vi "Set Modulation Mode.vi"(8 "error in (no error)":errorcluster, 9 "Modulation Mode (def: AM)":u16(ring)=1 items=["n/a", "AM", "FM", "PM", "FSK", "PWM"], 10 "Channel (0: Channel 1)":T1 items=["Channel 1", "Channel 2"], 11 "VISA resource name":refnum<visa-resource-name>) -> (0 "error out":errorcluster, 3 "VISA resource name out":refnum<visa-resource-name>)   [LabVIEW 2017, in "Tektronix AFG 3000 Series.lvlib"]
doc: "If pulse waveform and something other than PWM is desired, it will set the waveform to sine."
uses:
  Tektronix AFG 3000 Series.lvlib
  controls.llb/Channel.ctl
  controls.llb/Waveform Shape.ctl
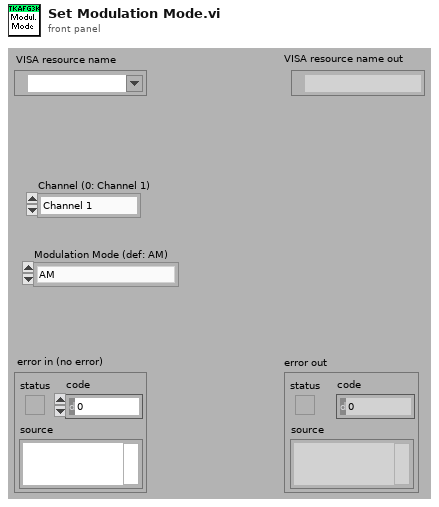
[diagram p1: front panel]
types:
  T1 = typedef "Channel.ctl" = u16
  T2 = typedef "Waveform Shape.ctl" = u16
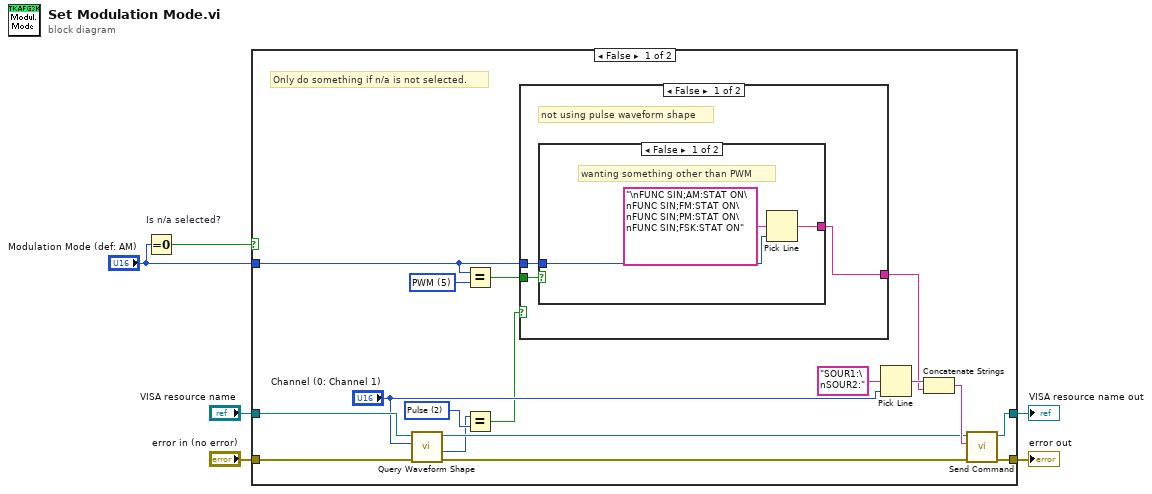
[diagram p0: block diagram]
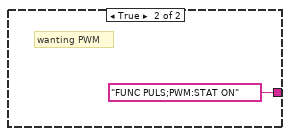
[diagram p2: hidden frame]
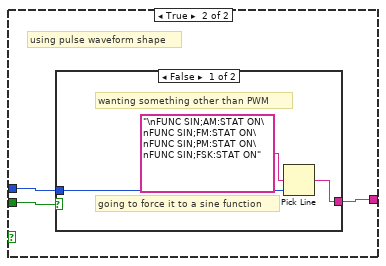
[diagram p3: hidden frame]
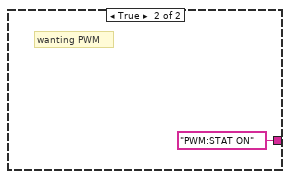
[diagram p4: hidden frame]
diagram:
  n1 = Equal To 0? "Is n/a selected?"(x="Modulation Mode (def: AM)") -> (x = 0?=w6:bool)
  n2 = case shown="False" w6 {
    tunnel: "Modulation Mode (def: AM)" -> [w7 _]
    tunnel: "error in (no error)" -> [w16 w38]
    tunnel: [w20 w38] -> w3
    tunnel: [w19 w39] -> w2
    tunnel: "VISA resource name" -> [w18 w39]
    frame False {
      w11 = u16 5 items=["n/a", "AM", "FM", "PM", "FSK", "PWM"] ("Modulation Mode (def: AM)")
      w13 = T2 2 items=["Sinusoid", "Square", "Pulse", "Ramp", "PRNoise", "DC", "SINC", "Gaussian", "Lorentz", "ERise", "EDecay", "Haversine", "User 1", "User 2", "User 3", "User 4", "EMemory", "EFile"] ("Waveform Shape")
      # "Only do something if n/a is not selected."
      n3 = call "Query Waveform Shape.vi"("error in (no error)"=w16, "Channel (0: Channel 1)"="Channel (0: Channel 1)", "VISA resource name"=w18) -> ("error out"=w15:errorcluster, "Waveform Shape"=w12:T2, "VISA resource name out"=w17:refnum<visa-resource-name>)  [unwired: 6 out]
      n4 = Equal?(x=w7, y=w11) -> (x = y?=w9:bool)
      n5 = Equal?(x=w12, y=w13) -> (x = y?=w10:bool)
      n6 = case shown="False" w10 {
        tunnel: w9 -> [w24 w33]
        tunnel: [w25 w32] -> w8
        tunnel: w7 -> [w26 w31]
        frame False {
          # "not using pulse waveform shape"
          n7 = case shown="False" w24 {
            tunnel: [w28 "FUNC PULS;PWM:STAT ON" ("format string")] -> w25
            tunnel: w26 -> [w27 _]
            frame False {
              # "wanting something other than PWM"
              n8 = Pick Line(multi-line string="\nFUNC SIN;AM:STAT ON\nFUNC SIN;FM:STAT ON\nFUNC SIN;PM:STAT ON\nFUNC SIN;FSK:STAT ON" ("format string"), line index=w27) -> (output string=w28:string)  [unwired: 1 out]
            }
            frame True {
              # "wanting PWM"
            }
          }
        }
        frame True {
          # "using pulse waveform shape"
          n9 = case shown="False" w33 {
            tunnel: [w35 "PWM:STAT ON" ("format string")] -> w32
            tunnel: w31 -> [w34 _]
            frame False {
              # "going to force it to a sine function"
              # "wanting something other than PWM"
              n10 = Pick Line(multi-line string="\nFUNC SIN;AM:STAT ON\nFUNC SIN;FM:STAT ON\nFUNC SIN;PM:STAT ON\nFUNC SIN;FSK:STAT ON" ("format string"), line index=w34) -> (output string=w35:string)  [unwired: 1 out]
            }
            frame True {
              # "wanting PWM"
            }
          }
        }
      }
      n11 = Pick Line(multi-line string="SOUR1:\nSOUR2:" ("string (\"\")"), line index="Channel (0: Channel 1)") -> (output string=w22:string)  [unwired: 1 out]
      n12 = Concatenate Strings(w22, w8) -> (w23:string)
      n13 = call "Send Command.vi"("error in (no error)"=w15, "write buffer"=w23, "VISA resource name"=w17) -> ("error out"=w20:errorcluster, "VISA resource name out"=w19:refnum<visa-resource-name>)  [unwired: 7 out]
    }
    frame True {
    }
  }
  "error out" <- w3
  "VISA resource name out" <- w2
